vi "RichToFlatnidevice_grpc_UnreserveResponse.vi"(5 "OutputClusterType":T1, 11 "InputCluster":T2) -> (3 "OutputCluster":T1)   [LabVIEW 2021, in "NI DAQmx_server.lvlib"]
uses:
  NI DAQmx_server.lvlib
  nidevice_grpc_UnreserveResponse.ctl
  nidevice_grpc_UnreserveResponse_Flat.ctl
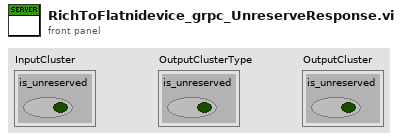
[diagram p1: front panel]
types:
  T1 = typedef "NI DAQmx_server.lvlib/nidevice_grpc_UnreserveResponse_Flat.ctl" = cluster{"is_unreserved":bool}
  T2 = typedef "NI DAQmx_server.lvlib/nidevice_grpc_UnreserveResponse.ctl" = cluster{"is_unreserved":bool}
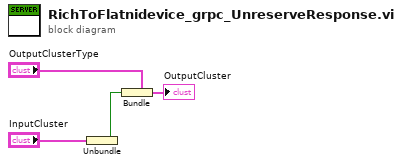
[diagram p0: block diagram]
diagram:
  n1 = Unbundle "Unbundle"("InputCluster") -> ("is_unreserved"=w1:bool)
  n2 = Bundle "Bundle"(cluster="OutputClusterType", "is_unreserved"=w1) -> (→"OutputCluster":T1)
